vi "Reaction Time.vi"() -> ()   [LabVIEW 2017]
panel:
  out "Reaction Time (ms)":dbl
  in  "stop":bool
  out "Square LED":bool
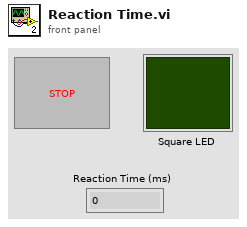
[diagram p1: front panel]
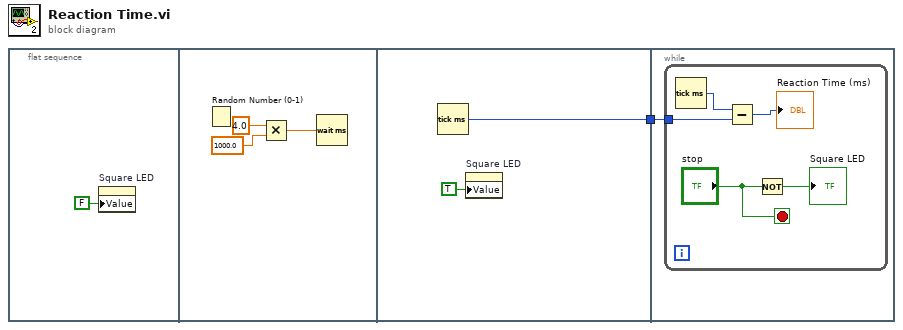
[diagram p0: block diagram]
diagram:
  n1 = flat-sequence {
    tunnel: [w6] -> w1
    tunnel: w1 -> [w8]
    frame #0 {
      n2 = property on="Square LED" class="Bool (strict)"("Value"=FALSE ("Square LED")) -> ()  [unwired: 2 in, 2 out]
    }
    frame #1 {
      n3 = Random Number (0-1)() -> ()  [unwired: 1 out]
      n4 = Multiply(x=4.0, y=1000.0) -> (x*y=w4:dbl)
      n5 = Wait (ms)(milliseconds to wait=w4) -> ()  [unwired: 1 out]
    }
    frame #2 {
      n6 = Tick Count (ms)() -> (millisecond timer value=w6:u32)
      n7 = property on="Square LED" class="Bool (strict)"("Value"=TRUE ("Square LED")) -> ()  [unwired: 2 in, 2 out]
    }
    frame #3 {
      n8 = while {
        tunnel: w8 -> [w12]
        stop <- "stop" stop-if-true
        n9 = Tick Count (ms)() -> (millisecond timer value=w13:u32)
        n10 = Subtract(x=w13, y=w12) -> (x-y=→"Reaction Time (ms)":u32)
        n11 = Not(x="stop") -> (.not. x?=→"Square LED":bool)
      }
    }
  }
